vi "AK Befehl Auswerten - AVL Sesam.vi"(10 "Array":string[](array[string])) -> (2 "String für schreiben":string)   [LabVIEW 2020, in "AK-Schnittstelle.lvlib"]
uses:
  AK-Schnittstelle.lvlib
  Aktionen Stoernummern pruefen.ctl
  Aktionen Zustandsfehlerinformation.ctl
  Seiten/FT-IR/FGV FT-IR Diagnose Aktionen.ctl
  Aktionen Gespeicherte Werte.ctl
  Funktionstasten/Funktionstasten-Aktion.ctl
  AK Namen Aktionen.ctl
  Seiten/System Einstellungen V2/Aktioen FGV System.ctl
  EPA 1065/Dichtheitstest 1065-345/Aktion Protokolldaten_Leak check.ctl
  Seiten/FT-IR/Aktion FGV Rezepte wechseln.ctl
  Seiten/FT-IR/FGV FT-IR Aktionen.ctl
  Schedule Modul/Aktion FGV Scheduler Status.ctl
  Seiten/System Einstellungen V2/Aktioen FGV System Konstanten.ctl
  Seiten/FT-IR/AK-manuell.ctl
  Funktionstasten/Zustaende.ctl
  Funktionstasten/Betriebsart.ctl
  EPA 1065/Dichtheitstest 1065-345/Aktion FGV Automatic start.ctl
  Bildwechsel/Bild-Auswahl.ctl
  Seiten/Log Konfig/Aktionen Trigger.ctl
  Seiten/FT-IR/TOOLweb Interface Library/TOOLweb Rezept wechseln.vi
  Funktionstasten/Funktionstasten.lvlib
  Seiten/Log Konfig/LogKonfig.lvlib
  Seiten/FT-IR/FT-IR.lvlib
  Seiten/FT-IR/FGV FT-IR Gasliste Aktionen.ctl
  Seiten/Erweiterte Konfig/Erweiterte Konfig.lvlib
  cRIO/PC/Kommunikation mit cRIO.lvlib
  Seiten/System Einstellungen V2/System Einstellungen V2.lvlib
  Allgemein/allgemeine Sub-VIs.lvlib
  Messdaten/Aktionen FGV Messdaten.ctl
  Messdaten/Messdaten.lvlib
  Schedule Modul/Schedule Modul.lvlib
  EPA 1065/Dichtheitstest 1065-345/Dichtheitstest 1065-345.lvlib
  Seiten/FT-IR/TOOLweb Interface Library/TOOLweb Interface.lvlib
  Bildwechsel/Bildwechsel.lvlib
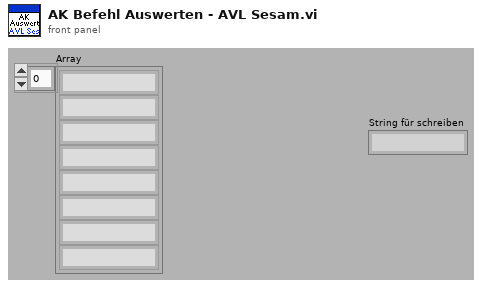
[diagram p1: front panel]
types:
  T1 = typedef "AK-Schnittstelle.lvlib/Aktionen Stoernummern pruefen.ctl" = enum16{"lesen", "prüfen"}
  T2 = typedef "AK-Schnittstelle.lvlib/Aktionen Zustandsfehlerinformation.ctl" = enum16{"OK", "Offline", "Busy", "Syntax Error", "Datenfehler"}
  T3 = typedef "AK-Schnittstelle.lvlib/Aktionen Gespeicherte Werte.ctl" = enum16{"lesen", "laden", "speichern", "Seriell", "TCP", "Diverse", "AKTIV", "AK-Namen"}
  T4 = typedef "FT-IR.lvlib/FGV FT-IR Diagnose Aktionen.ctl" = enum16{"Lesen", "Diagnose Schreiben", "Min Schreiben", "Max Schreiben"}
  T5 = typedef "Funktionstasten.lvlib/Funktionstasten-Aktion.ctl" = enum16{"Initialisieren", "Zustand setzen", "Taste gedrückt", "Fehler speichern", "Lesen", "Manuell", "Remote", "Bitparallel", "Samplepoint", "Zeit Prüfen", "reset Umschalten"}
  T6 = typedef "AK-Schnittstelle.lvlib/AK Namen Aktionen.ctl" = enum16{"lesen", "laden", "speichern Namen", "AK Namen", "Liste erstellen", "EKFG erstellen", "speichern EKFG", "EKFG schreiben", "Neuen Eintrag erzeugen"}
  T7 = typedef "FT-IR.lvlib/FGV FT-IR Gasliste Aktionen.ctl" = enum16{"lesen", "Gasliste FT-IR", "Gasliste ausgelesen", "laden", "speichern", "löschen"}
  T8 = typedef "System Einstellungen V2.lvlib/Aktioen FGV System.ctl" = enum16{"lesen", "laden", "speichern", "Optionen schreiben", "Zeitstempel", "Reset BMP", "Reset SQP", "Wartung", "Werkseinstellung"}
  T9 = typedef "Messdaten.lvlib/Aktionen FGV Messdaten.ctl" = enum16{"lesen", "schreiben", "löschen", "Mittelwerte", "Komponente"}
  T10 = typedef "EPA 1065.lvlib/Dichtheitstest 1065-345.lvlib/Aktion Protokolldaten_Leak check.ctl" = enum16{"lesen", "Zeitstempel", "Bearbeiter", "Daten", "Auswertung", "löschen"}
  T11 = typedef "FT-IR.lvlib/FGV FT-IR Aktionen.ctl" = enum16{"lesen", "NOG setzen", "NOS setzen", "Initialisieren", "speichern", "ALLES setzen", "FT-IR Spektrum loggen", "Komm Stoppen", "Spektrum LogKonfig"}
  T12 = typedef "FT-IR.lvlib/Aktion FGV Rezepte wechseln.ctl" = enum16{"lesen", "Rezepte", "Rezeptindex", "Diesel", "Gasoline", "NCG", "laden", "speichern", "AK/Man"}
  T13 = typedef "Schedule Modul.lvlib/Aktion FGV Scheduler Status.ctl" = enum16{"lesen", "init", "aktiv", "inaktiv"}
  T14 = typedef "System Einstellungen V2.lvlib/Aktioen FGV System Konstanten.ctl" = enum16{"lesen", "laden", "speichern", "Sprache"}
  T15 = typedef "FT-IR.lvlib/AK-manuell.ctl" = enum16{"manuell", "Diesel", "CNG", "Gasoline"}
  T16 = typedef "Funktionstasten.lvlib/Zustaende.ctl" = enum16{"Standby", "Pause", "Eco", "Messen", "Kalibrieren", "Spülen Filter", "Spülen Leitung", "Umgebungsluft", "0-Gas", "Cal-Gas", "CG zu PNS", "-------------", "Init 1", "Init 2", "Init 3", "Init 4", "Messen vorbereiten", "Messen durchführen", "Exit"}
  T17 = typedef "Funktionstasten.lvlib/Betriebsart.ctl" = enum16{"Manuell", "Remote", "Bitparallel"}
  T18 = typedef "EPA 1065.lvlib/Dichtheitstest 1065-345.lvlib/Aktion FGV Automatic start.ctl" = enum16{"lesen", "Test starten aktiv", "Test starten inaktiv", "Seite merken", "Seite zurücksetzen", "AK Start inaktiv"}
  T19 = typedef "Bildwechsel.lvlib/Bild-Auswahl.ctl" = enum16{"lesen", "Initialisieren", "Beenden", "Grafik", "Anlagenübersicht", "Anlagengrenzwerte", "Log Konfig", "Gaszuordnung AO", "Erw. Konfiguration", "FT-IR  ", "Störmeldungen", "Störmeldepuffer", "Störmeldekonfig", "PNS Grenzwerte", "Statusübersicht", "Linearisierung", "ARN", "EPA Dichtheitstest", "FID", "PMA", "CalGas", "Lambda", "Interference", "Amium PNS", "EPA T90", "Interference N2O", "Scheduler", "Systemeinstellungen", "EPA Drift", "CAN Konfig"}
  T20 = typedef "LogKonfig.lvlib/Aktionen Trigger.ctl" = enum16{"lesen", "ALLE schreiben", "Trigger prüfen", "Trigger rücksetzen"}
  T21 = typedef "AK-Schnittstelle.lvlib/Diverse gespeicherte Werte.ctl" = cluster{"Kalibriergaseingang":i16, "SamplePoint":i16, "CalGas zu PNS":i16, "Gas-Reihenfolge":i16[], "Zeit 0-Gas":sgl, "Zeit CalGas":sgl, "AK Befehlssatz":T22}
  T22 = typedef "AK-Schnittstelle.lvlib/AK Befehlssatz.ctl" = enum16{"MEXA", "IAG v1.4", "AVL (Puma)", "PEUS"}
  T23 = typedef "Verwaltung - cRIO.lvlib/Analog Eingaenge.ctl" = cluster{"AI0: Durchfluss FT-IR":sgl, "AI1: Druck Ausgang":sgl, "AI2: Umgebungsdruck":sgl, "AI3: Druck FT-IR":sgl, "AI4: Druck CalGas":sgl, "AI5: Reserve":sgl, "AI6: Reserve":sgl, "AI7: Reserve":sgl, "Rohwert Durchfluss FT-IR":sgl, "Rohwert Druck Ausgang":sgl, "Rohwert Umgebungsdruck":sgl, "Rohwert Druck FT-IR":sgl, "Rohwert Druck CalGas":sgl, "Rohwert AI5":sgl, "Rohwert AI6":sgl, "Rohwert AI7":sgl, "Rohwert Diffdruck mbar FTIR":sgl}
  T24 = typedef "String - Ausgabefeld.ctl" = string
  T25 = typedef "System Einstellungen V2.lvlib/Optionen.ctl" = cluster{"Störmeldep.":bool, "Betriebszustände":bool, "AK in ppm":bool, "log Cal-Gas":bool, "log 0-Gas":bool, "Durchflusssensor 0-5V":bool, "PNS?":bool, "Mit N2 spülen":bool, "TRE08":bool, "Amium 10-Fach":bool, "Verticale Scrollbar aktiv":bool, "Loggingtakt":bool, "AK Rezeptwechsel gleich wie MKS":bool, "NG ECO":bool}
  T26 = typedef "EPA 1065.lvlib/Dichtheitstest 1065-345.lvlib/Leak Daten.ctl" = cluster{"Gesamtes Volumen":sgl, "p 1":sgl, "p 2":sgl, "T 1":sgl, "T 2":sgl, "t 1":timestamp, "t 2":timestamp, "Ergebnis mol/s":sgl, "Grenze mol/s":sgl, "Leak in %":sgl, "Ergebnis mbar":sgl, "Grenze mbar":sgl}
  T27 = typedef "Verwaltung - cRIO.lvlib/TC Eingaenge.ctl" = cluster{"TC0: Reserve":sgl, "TC1: HL zu FT-IR":sgl, "TC2: HL Extern SP1":sgl, "TC3: HL Extern SP2":sgl, "TC4: Reserve":sgl, "TC5: Reserve":sgl, "TC6: Reserve":sgl, "TC7: Reserve":sgl, "TC8: FT-IR":sgl, "TC9: Reserve":sgl, "TC10: Schaltschrank":sgl, "TC11: Umgebung":sgl}
  T28 = cluster{"Modell":string, "ProjektNummer":string, "Software Version":string, "Seriennummer":string}
  T29 = typedef "LogKonfig.lvlib/Element Triggerereignisse.ctl" = cluster{"Trigger verwenden":T30, "Messwert":u16, "kl./gr.":u16, "Wert":sgl, "Puffergröße":sgl}
  T30 = typedef "LogKonfig.lvlib/Auswahlfeld aktiviert-deaktiviert.ctl" = u16
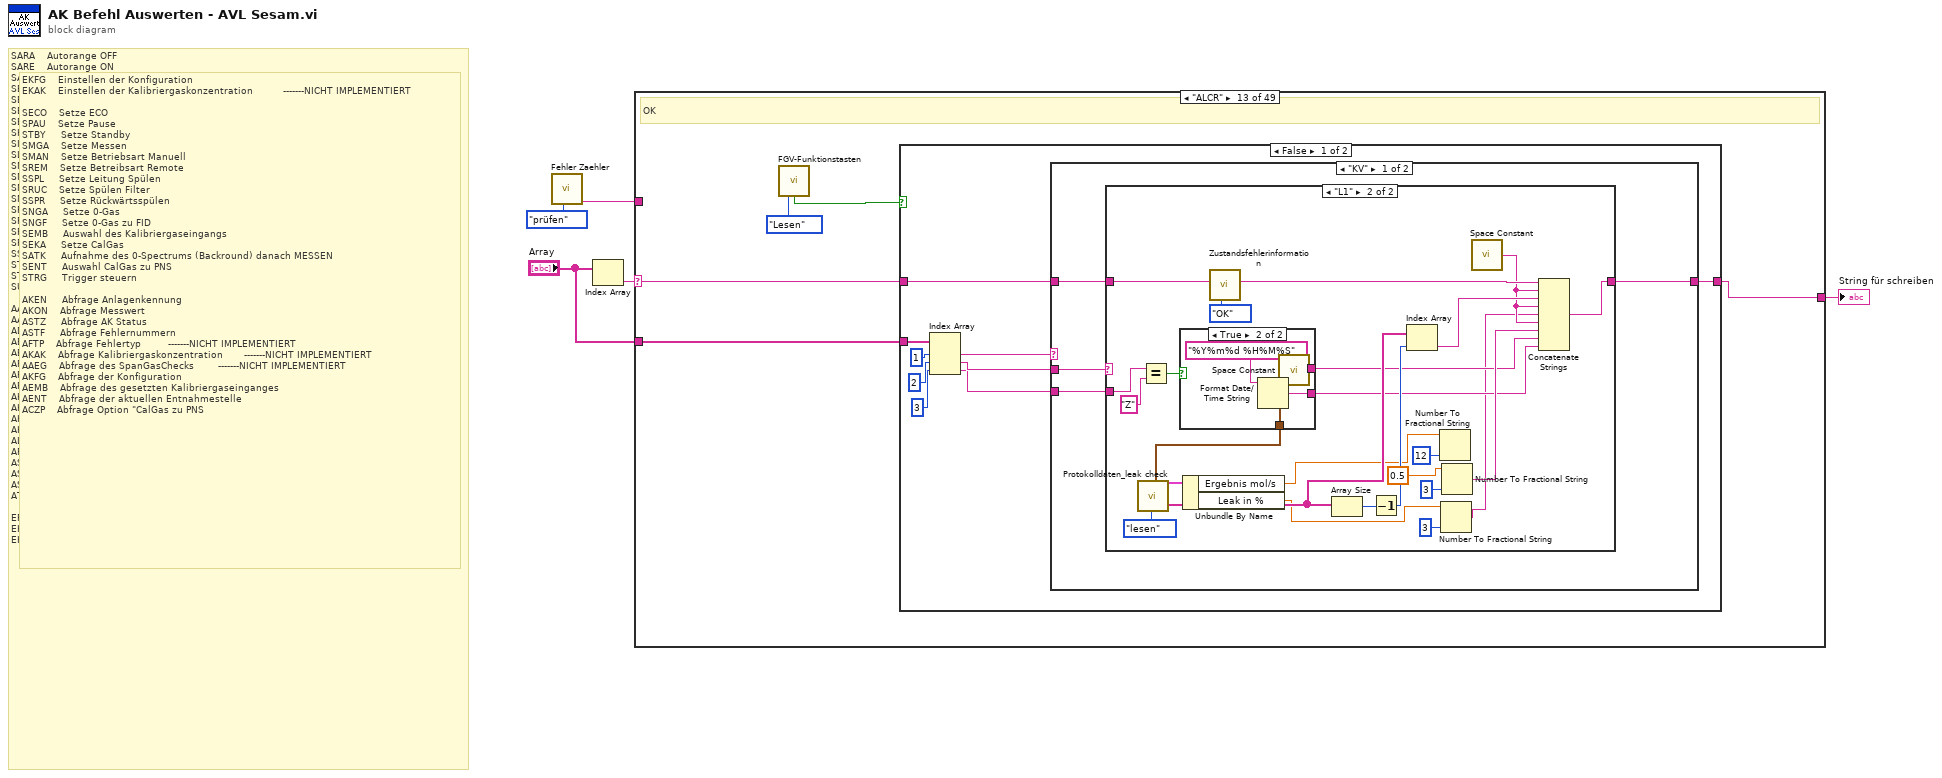
[diagram p0: block diagram]
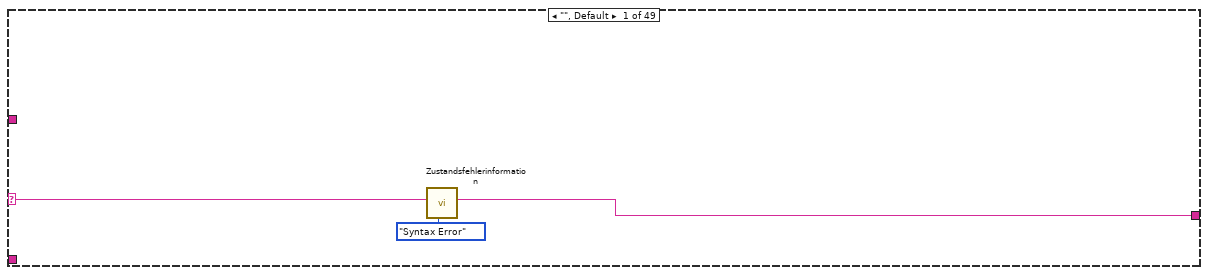
[diagram p2: hidden frame]
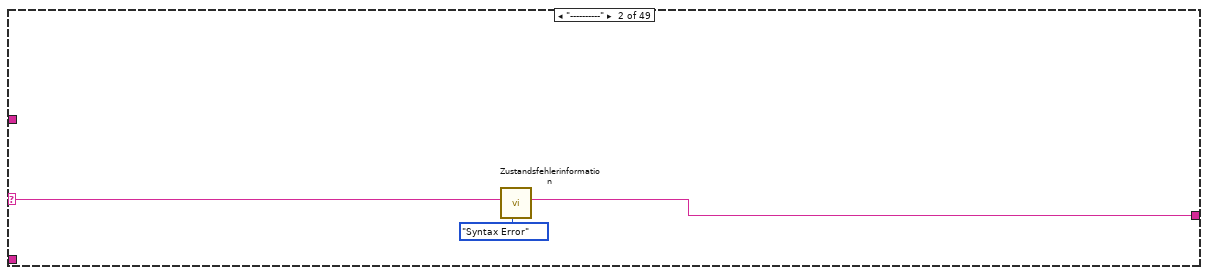
[diagram p3: hidden frame]
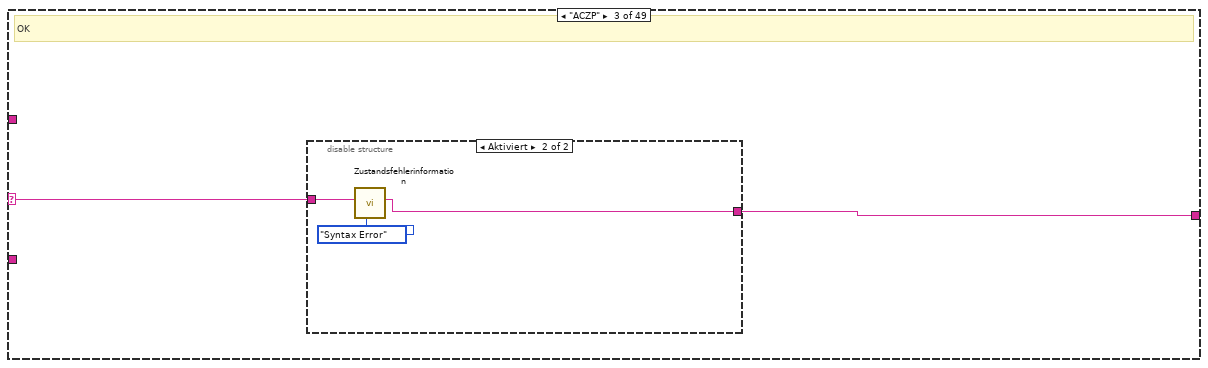
[diagram p4: hidden frame]
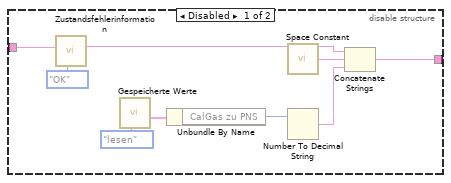
[diagram p5: hidden frame]
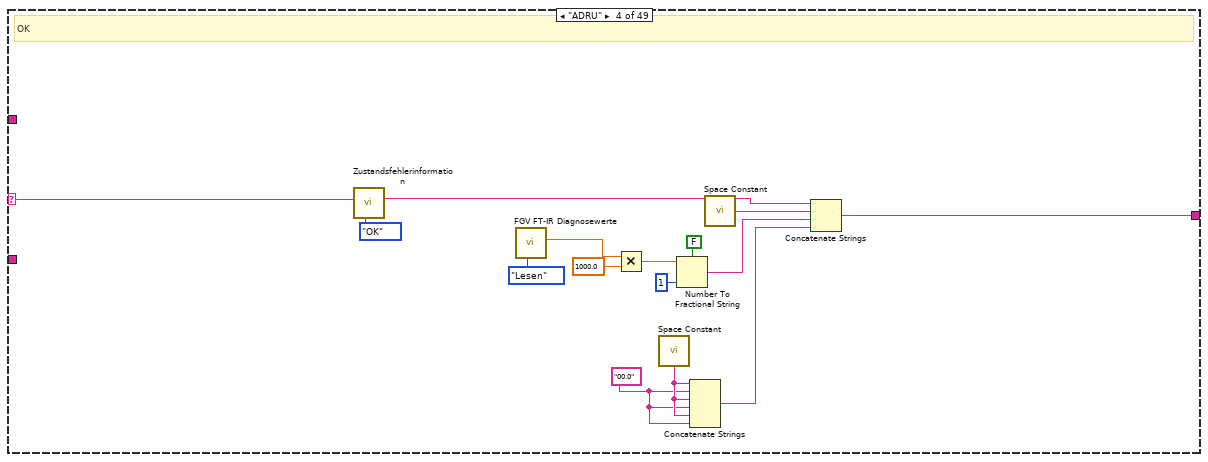
[diagram p6: hidden frame]
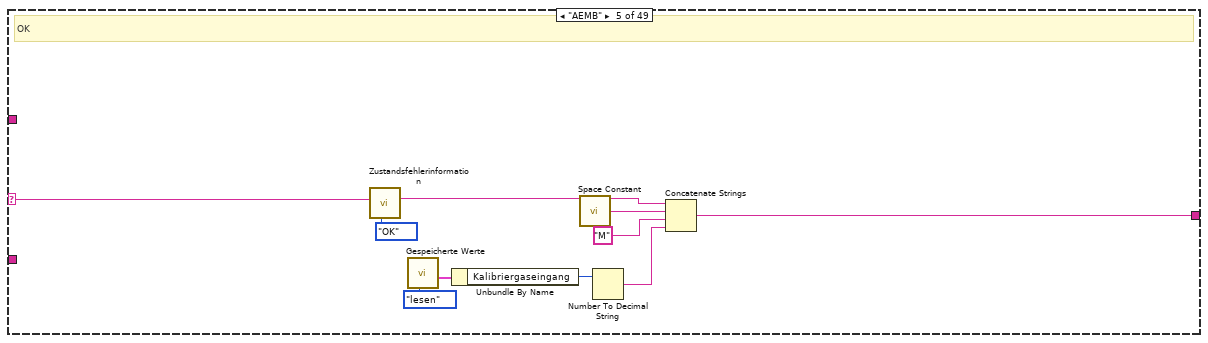
[diagram p7: hidden frame]
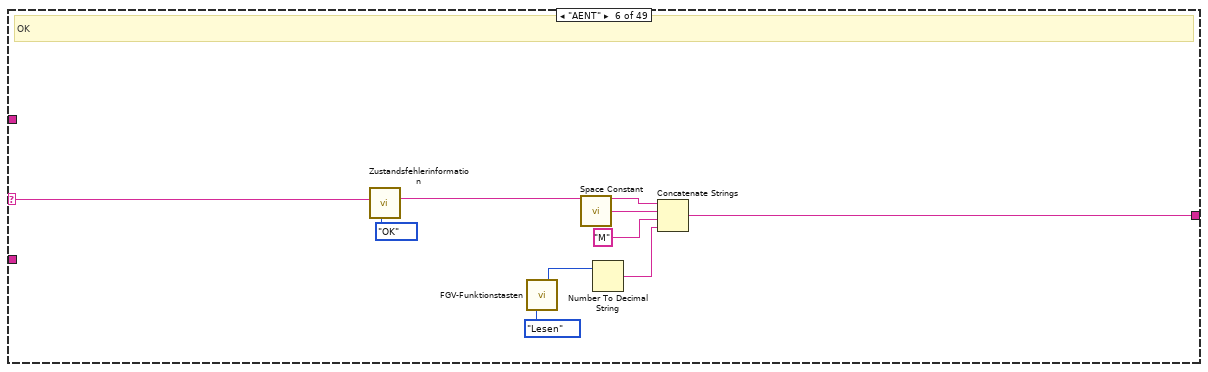
[diagram p8: hidden frame]
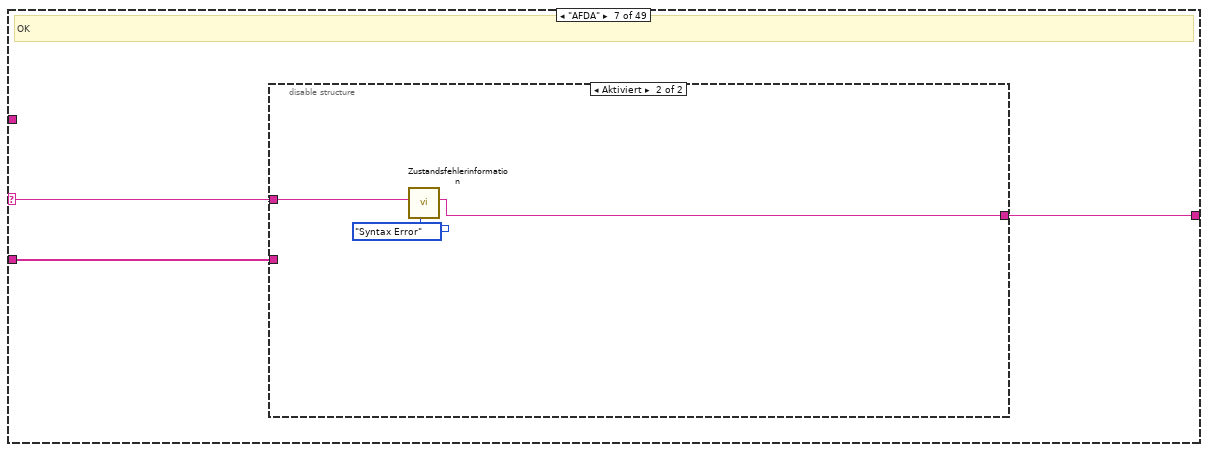
[diagram p9: hidden frame]
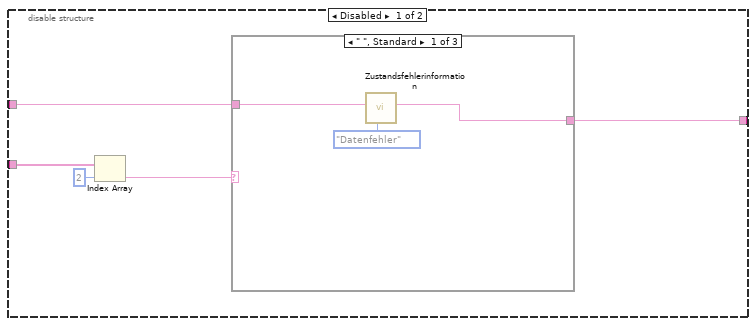
[diagram p10: hidden frame]
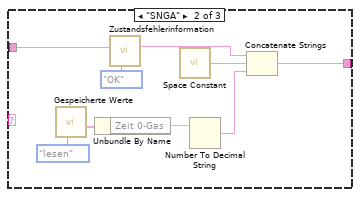
[diagram p11: hidden frame]
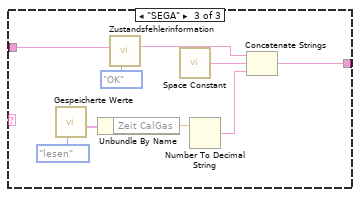
[diagram p12: hidden frame]
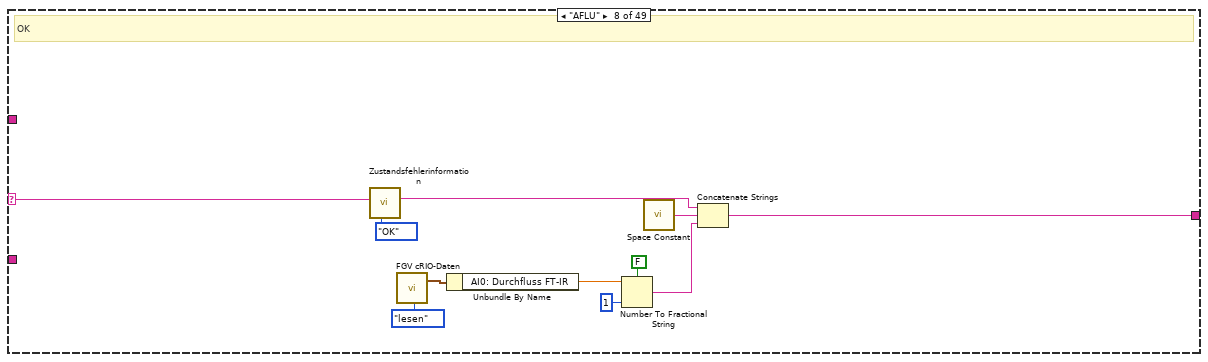
[diagram p13: hidden frame]
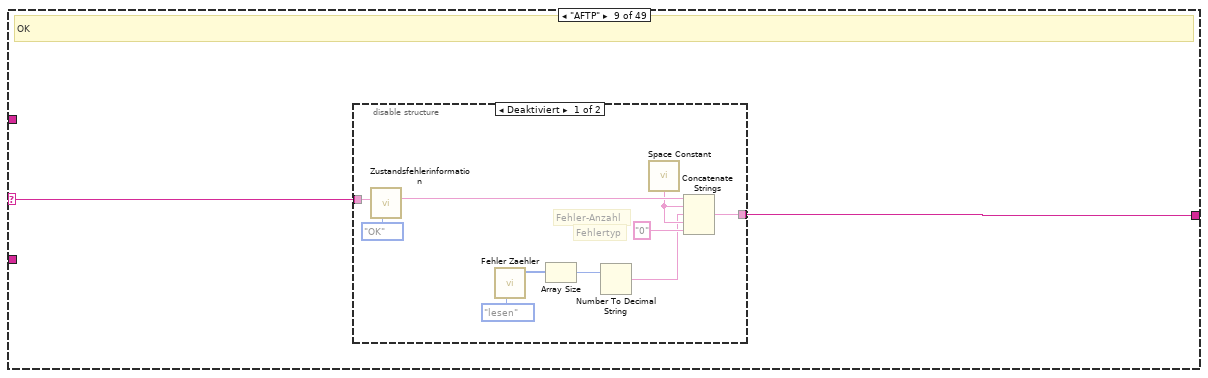
[diagram p14: hidden frame]
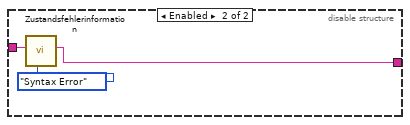
[diagram p15: hidden frame]
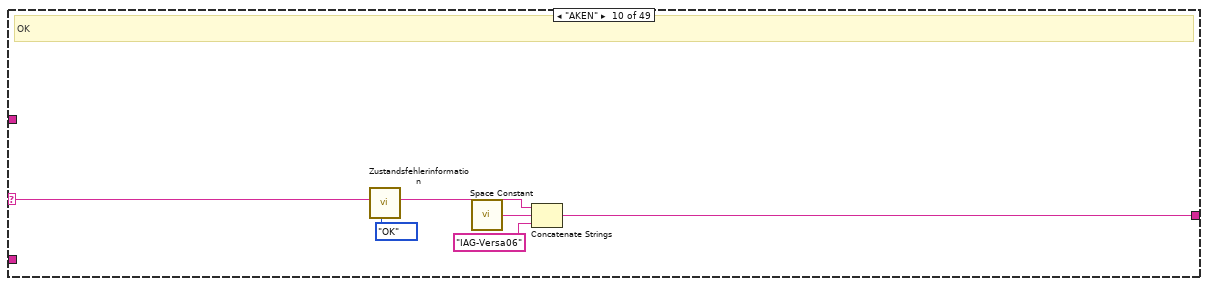
[diagram p16: hidden frame]
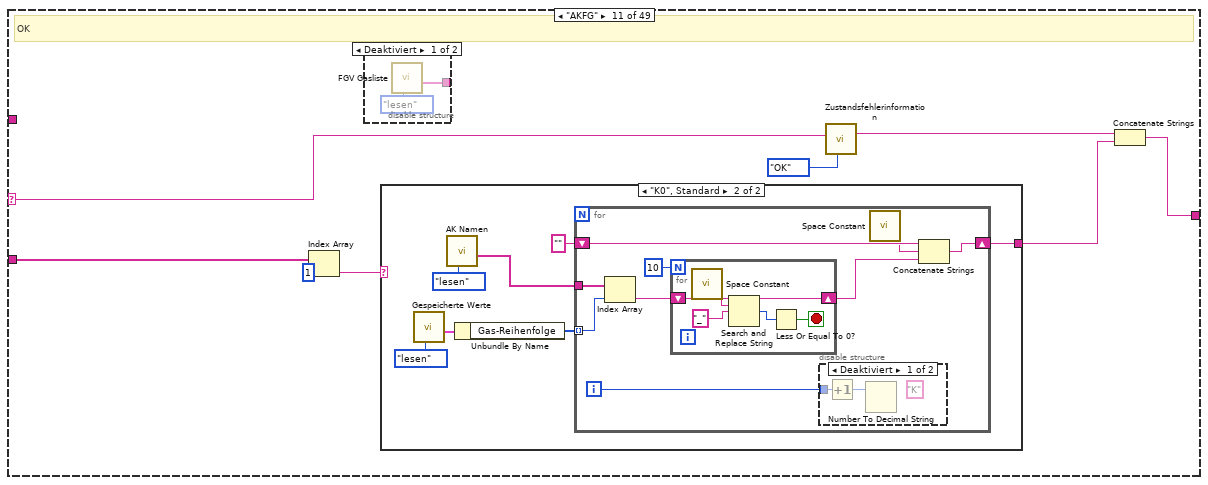
[diagram p17: hidden frame]
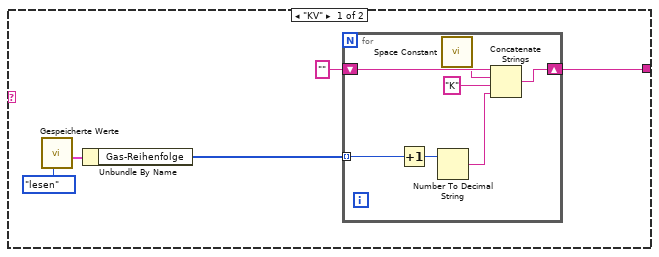
[diagram p18: hidden frame]
diagram:
  # "SARA    Autorange OFF\nSARE    Autorange ON\nSATK    Zero / Span Adjust\nSEGA    Apply Span Gas\nSEKA    Performing FTIR Span Gas Check\nSEMB    Selecting Calibration Gas Inlet\nSENT    Set Sampling\nSHUP    Hang-Up Test         -------NICHT IMPLEMENTIERT\nSINT     Starting Continous FTIR Measurement\nSLEC     Leak Check\nSMAN    Set Manual\nSMGA    Set Measure\nSNGA    Apply Zero Gas\nSNKA    Adjust Zero Point\nSPAU    Pause Modus\nSREM    Set Remote\nSRES    Set Reset\nSRUC / SRUK  Backflush\nSSPL     Purge Gas Lines\nSTBY    Set Standby\nSTUN    Automatically Adjusting Optics and Signals         -------NICHT IMPLEMENTIERT\nSUGR    Recording Zero Energy Spectrum\n\nAAEG    Inquire Span Point Deviation\nAANG    Inquire Zero Point Deviation\nADRU    Inquire Pressure of SESAM FTIR\nAENT    Inquire Sampling Points\nAEMB    Inquire Measuring Range\nAFDA    Inquire Function Duration\nAFLU     Inquire Sample Flow of SBEAM FTIR\nAFTP     Inquire Error Type\nAHUP    Inquire Hangup Result         -------NICHT IMPLEMENTIERT\nAKAK    Inquire Span Gas Concentrations         -------NICHT IMPLEMENTIERT\nAKFG    Inquire Configuration\nAKON   Inquire Measuring Value\nALEC    Inquire Leak Check Result         -------NICHT IMPLEMENTIERT\nAREG    Inquire Control Variable of SESAM FTIR          -------NICHT IMPLEMENTIERT\nASTA    Inquire Erroneous Channel         -------NICHT IMPLEMENTIERT\nASTF    Inquire Error Numbers\nASTZ    Inquire AK Status\nATEM   Inquire Temperature of SESAM FTIR\n\nEFDA   Configure Function Duration\nEKAK   Configure Span Gas Concentration         -------NICHT IMPLEMENTIERT\nEKFG   Configure Configuration"
  # "EKFG    Einstellen der Konfiguration\nEKAK    Einstellen der Kalibriergaskonzentration          -------NICHT IMPLEMENTIERT\n\nSECO    Setze ECO\nSPAU    Setze Pause\nSTBY     Setze Standby\nSMGA    Setze Messen\nSMAN    Setze Betriebsart Manuell\nSREM    Setze Betreibsart Remote\nSSPL     Setze Leitung Spülen\nSRUC    Setze Spülen Filter\nSSPR     Setze Rückwärtsspülen\nSNGA     Setze 0-Gas\nSNGF     Setze 0-Gas zu FID\nSEMB     Auswahl des Kalibriergaseingangs\nSEKA     Setze CalGas\nSATK     Aufnahme des 0-Spectrums (Backround) danach MESSEN\nSENT     Auswahl CalGas zu PNS\nSTRG     Trigger steuern\n\nAKEN     Abfrage Anlagenkennung\nAKON    Abfrage Messwert\nASTZ     Abfrage AK Status\nASTF     Abfrage Fehlernummern\nAFTP    Abfrage Fehlertyp         -------NICHT IMPLEMENTIERT\nAKAK    Abfrage Kalibriergaskonzentration       -------NICHT IMPLEMENTIERT\nAAEG    Abfrage des SpanGasChecks        -------NICHT IMPLEMENTIERT\nAKFG    Abfrage der Konfiguration\nAEMB    Abfrage des gesetzten Kalibriergaseinganges\nAENT    Abfrage der aktuellen Entnahmestelle\nACZP    Abfrage Option \"CalGas zu PNS"
  n1 = call "Fehler Zaehler.vi"("Aktionen"=Aktionen_Stoernummern_pruefen."prüfen") -> ("Fehlerzähler"=w3:string)  [unwired: 7 in, 3 out]
  n2 = Index Array(array="Array") -> (element=w2:string)  [unwired: 1 in]
  n3 = case shown="\"ALCR\"" w2 {
    selector: w2 -> [w7 w10 w12 w38 w48 w57 w61 w100 w103 w120 w129 w189 w245 w317 w321 w342 w349 w367 w407 w432 w437 w475 w506 w541 w544 w547 w551 w553 w567 w571 w593 w620 w623 w659 w662 w676 w679 w683 w685 w689 w691 w695 w706 w716 w726 w730 w733 w736 w758]
    tunnel: [w6 w9 w13 w40 w50 w59 w62 w102 w104 w122 w131 w190 w242 w319 w320 w344 w351 w365 w409 w434 w436 w474 w505 w540 w543 w546 w550 w552 w566 w570 w592 w619 w622 w658 w661 w675 w678 w682 w684 w688 w690 w694 w705 w715 w725 w729 w732 w735 w757] -> w5
    tunnel: w3 -> [_ _ _ _ _ _ _ _ _ _ _ _ _ _ _ _ _ _ _ _ _ _ _ _ _ _ _ _ _ _ _ _ _ _ _ _ _ _ _ _ _ _ _ _ _ _ _ _ _]
    tunnel: "Array" -> [_ _ _ _ _ _ w60 _ _ _ w126 w183 w241 _ _ _ _ w366 _ _ w435 w476 w507 _ _ _ _ _ _ w569 w591 _ w630 _ _ _ _ _ _ _ _ _ w698 w707 w718 _ _ w734 _]
    frame "", Default {
      n4 = call "Zustandsfehlerinformation.vi"("Aktionen"=Aktionen_Zustandsfehlerinformation."Syntax Error", "String"=w7) -> ("String"=w6:string)  [unwired: 9 in]
    }
    frame "----------" {
      n5 = call "Zustandsfehlerinformation.vi"("Aktionen"=Aktionen_Zustandsfehlerinformation."Syntax Error", "String"=w10) -> ("String"=w9:string)  [unwired: 9 in]
    }
    frame "ACZP" {
      # "OK"
      n6 = disable-structure shown="Aktiviert" {
        disable-tunnel: [w22 w23] -> w13
        disable-tunnel: w12 -> [w20 w24]
        frame Disabled {
          n7 = call "Zustandsfehlerinformation.vi"("Aktionen"=Aktionen_Zustandsfehlerinformation."OK", "String"=w20) -> ("String"=w19:string)  [unwired: 9 in]
          n8 = call "Gespeicherte Werte.vi"("Aktionen"=Aktionen_Gespeicherte_Werte."lesen") -> ("Diverse Werte"=w14:T21)  [unwired: 6 in, 4 out]
          n9 = Unbundle By Name(w14) -> ("CalGas zu PNS"=w17:i16)
          n10 = call <vilib>:"Space Constant.vi"() -> ("String"=w15:string)
          n11 = Number To Decimal String(number=w17) -> (decimal integer string=w16:string)  [unwired: 1 in]
          n12 = Concatenate Strings(w19, w15, w16) -> (w22:string)
        }
        frame Enabled {
          n13 = call "Zustandsfehlerinformation.vi"("Aktionen"=Aktionen_Zustandsfehlerinformation."Syntax Error", "String"=w24) -> ("String"=w23:string)  [unwired: 9 in]
        }
      }
    }
    frame "ADRU" {
      w27 = "00.0" ("String in F-Format")
      # "OK"
      n14 = call "Zustandsfehlerinformation.vi"("Aktionen"=Aktionen_Zustandsfehlerinformation."OK", "String"=w38) -> ("String"=w37:string)  [unwired: 9 in]
      n15 = call "FGV FT-IR Diagnosewerte.vi"("Aktionen"=FGV_FT-IR_Diagnose_Aktionen."Lesen") -> ("Druck"=w34:dbl)  [unwired: 5 in, 5 out]
      n16 = Multiply(x=w34, y=1000.0) -> (x*y=w31:dbl)
      n17 = call <vilib>:"Space Constant.vi"() -> ("String"=w28:string)
      n18 = Number To Fractional String(use system decimal point (T)=FALSE ("Systemdezimalzeichen verwenden (T)"), number=w31, precision (6)=i16 1 ("Genauigkeit (6)")) -> (F-format string=w29:string)  [unwired: 1 in]
      n19 = Concatenate Strings(w28, w27, w28, w27, w28, w27) -> (w26:string)
      n20 = call <vilib>:"Space Constant.vi"() -> ("String"=w36:string)
      n21 = Concatenate Strings(w37, w36, w29, w26) -> (w40:string)
    }
    frame "AEMB" {
      # "OK"
      n22 = call "Zustandsfehlerinformation.vi"("Aktionen"=Aktionen_Zustandsfehlerinformation."OK", "String"=w48) -> ("String"=w47:string)  [unwired: 9 in]
      n23 = call "Gespeicherte Werte.vi"("Aktionen"=Aktionen_Gespeicherte_Werte."lesen") -> ("Diverse Werte"=w41:T21)  [unwired: 6 in, 4 out]
      n24 = Unbundle By Name(w41) -> ("Kalibriergaseingang"=w45:i16)
      n25 = call <vilib>:"Space Constant.vi"() -> ("String"=w42:string)
      n26 = Number To Decimal String(number=w45) -> (decimal integer string=w43:string)  [unwired: 1 in]
      n27 = Concatenate Strings(w47, w42, "M" ("String"), w43) -> (w50:string)
    }
    frame "AENT" {
      # "OK"
      n28 = call "Zustandsfehlerinformation.vi"("Aktionen"=Aktionen_Zustandsfehlerinformation."OK", "String"=w57) -> ("String"=w56:string)  [unwired: 9 in]
      n29 = call "FGV-Funktionstasten.vi"("Aktion"=Funktionstasten-Aktion."Lesen") -> ("Samplepoint"=w51:u16)  [unwired: 7 in, 7 out]
      n30 = call <vilib>:"Space Constant.vi"() -> ("String"=w53:string)
      n31 = Number To Decimal String(number=w51) -> (decimal integer string=w54:string)  [unwired: 1 in]
      n32 = Concatenate Strings(w56, w53, "M" ("String"), w54) -> (w59:string)
    }
    frame "AFDA" {
      # "OK"
      n33 = disable-structure shown="Aktiviert" {
        disable-tunnel: [w67 w89] -> w62
        disable-tunnel: w61 -> [w66 w90]
        disable-tunnel: w60 -> [w65 _]
        frame Disabled {
          n34 = Index Array(array=w65, index=2 ("Index")) -> (element=w63:string)
          n35 = case shown="\" \", Standard" w63 {
            tunnel: [w68 w79 w88] -> w67
            tunnel: w66 -> [w69 w77 w86]
            frame " ", Default {
              n36 = call "Zustandsfehlerinformation.vi"("Aktionen"=Aktionen_Zustandsfehlerinformation."Datenfehler", "String"=w69) -> ("String"=w68:string)  [unwired: 9 in]
            }
            frame "SNGA" {
              n37 = call "Gespeicherte Werte.vi"("Aktionen"=Aktionen_Gespeicherte_Werte."lesen") -> ("Diverse Werte"=w74:T21)  [unwired: 6 in, 4 out]
              n38 = Unbundle By Name(w74) -> ("Zeit 0-Gas"=w72:sgl)
              n39 = call "Zustandsfehlerinformation.vi"("Aktionen"=Aktionen_Zustandsfehlerinformation."OK", "String"=w77) -> ("String"=w76:string)  [unwired: 9 in]
              n40 = call <vilib>:"Space Constant.vi"() -> ("String"=w75:string)
              n41 = Number To Decimal String(number=w72) -> (decimal integer string=w71:string)  [unwired: 1 in]
              n42 = Concatenate Strings(w76, w75, w71) -> (w79:string)
            }
            frame "SEGA" {
              n43 = call "Gespeicherte Werte.vi"("Aktionen"=Aktionen_Gespeicherte_Werte."lesen") -> ("Diverse Werte"=w83:T21)  [unwired: 6 in, 4 out]
              n44 = Unbundle By Name(w83) -> ("Zeit CalGas"=w81:sgl)
              n45 = call "Zustandsfehlerinformation.vi"("Aktionen"=Aktionen_Zustandsfehlerinformation."OK", "String"=w86) -> ("String"=w85:string)  [unwired: 9 in]
              n46 = call <vilib>:"Space Constant.vi"() -> ("String"=w84:string)
              n47 = Number To Decimal String(number=w81) -> (decimal integer string=w80:string)  [unwired: 1 in]
              n48 = Concatenate Strings(w85, w84, w80) -> (w88:string)
            }
          }
        }
        frame Enabled {
          n49 = call "Zustandsfehlerinformation.vi"("Aktionen"=Aktionen_Zustandsfehlerinformation."Syntax Error", "String"=w90) -> ("String"=w89:string)  [unwired: 9 in]
        }
      }
    }
    frame "AFLU" {
      # "OK"
      n50 = call "Zustandsfehlerinformation.vi"("Aktionen"=Aktionen_Zustandsfehlerinformation."OK", "String"=w100) -> ("String"=w99:string)  [unwired: 9 in]
      n51 = call "FGV cRIO-Daten.vi"("Aktion"=enum16{"lesen", "schreiben"}."lesen") -> ("Analog Input"=w96:T23)  [unwired: 9 in, 9 out]
      n52 = Unbundle By Name(w96) -> ("AI0: Durchfluss FT-IR"=w93:sgl)
      n53 = Number To Fractional String(use system decimal point (T)=FALSE ("Systemdezimalzeichen verwenden (T)"), number=w93, precision (6)=i16 1 ("Genauigkeit (6)")) -> (F-format string=w92:string)  [unwired: 1 in]
      n54 = call <vilib>:"Space Constant.vi"() -> ("String"=w98:string)
      n55 = Concatenate Strings(w99, w98, w92) -> (w102:string)
    }
    frame "AFTP" {
      # "OK"
      n56 = disable-structure shown="Deaktiviert" {
        disable-tunnel: [w114 w115] -> w104
        disable-tunnel: w103 -> [w112 w116]
        frame Disabled {
          # "Fehlertyp"
          # "Fehler-Anzahl"
          n57 = call "Zustandsfehlerinformation.vi"("Aktionen"=Aktionen_Zustandsfehlerinformation."OK", "String"=w112) -> ("String"=w111:string)  [unwired: 9 in]
          n58 = call "Fehler Zaehler.vi"("Aktionen"=Aktionen_Stoernummern_pruefen."lesen") -> ("Fehler Nummern"=w109:i32[])  [unwired: 7 in, 3 out]
          n59 = Array Size(array=w109) -> (size(s)=w108:i32)
          n60 = Number To Decimal String(number=w108) -> (decimal integer string=w105:string)  [unwired: 1 in]
          n61 = call <vilib>:"Space Constant.vi"() -> ("String"=w107:string)
          n62 = Concatenate Strings(w111, w107, w105, w107, "0" ("String")) -> (w114:string)
        }
        frame Enabled {
          n63 = call "Zustandsfehlerinformation.vi"("Aktionen"=Aktionen_Zustandsfehlerinformation."Syntax Error", "String"=w116) -> ("String"=w115:string)  [unwired: 9 in]
        }
      }
    }
    frame "AKEN" {
      # "OK"
      n64 = call "Zustandsfehlerinformation.vi"("Aktionen"=Aktionen_Zustandsfehlerinformation."OK", "String"=w120) -> ("String"=w119:string)  [unwired: 9 in]
      n65 = call <vilib>:"Space Constant.vi"() -> ("String"=w118:string)
      n66 = Concatenate Strings(w119, w118, "IAG-Versa06" ("String")) -> (w122:string)
    }
    frame "AKFG" {
      # "OK"
      n67 = Index Array(array=w126, index=1 ("Index")) -> (element=w124:string)
      n68 = disable-structure shown="Deaktiviert" {
        disable-tunnel: [w168 _] -> _
        frame Disabled {
          n69 = call "FGV Gasliste.vi"("Aktionen"=FGV_FT-IR_Gasliste_Aktionen."lesen") -> ("Aktuelle Gasliste gesamt"=w168:T24[])  [unwired: 8 in, 2 out]
        }
        frame Enabled {
        }
      }
      n70 = case shown="\"K0\", Standard" w124 {
        tunnel: [w132 w148] -> w127
        frame "KV" {
          n71 = call "Gespeicherte Werte.vi"("Aktionen"=Aktionen_Gespeicherte_Werte."lesen") -> ("Diverse Werte"=w136:T21)  [unwired: 6 in, 4 out]
          n72 = Unbundle By Name(w136) -> ("Gas-Reihenfolge"=w134:i16[])
          n73 = for {
            tunnel: w134 -> [w139] mode=indexing
            shift-right: [w143] -> w132
            shift-left: "" -> [w142]
            n74 = Increment(x=w139) -> (x+1=w140:i16)
            n75 = Number To Decimal String(number=w140) -> (decimal integer string=w137:string)  [unwired: 1 in]
            n76 = call <vilib>:"Space Constant.vi"() -> ("String"=w141:string)
            n77 = Concatenate Strings(w142, w141, "K" ("String"), w137) -> (w143:string)
          }
        }
        frame "K0", Default {
          n78 = call "Gespeicherte Werte.vi"("Aktionen"=Aktionen_Gespeicherte_Werte."lesen") -> ("Diverse Werte"=w146:T21)  [unwired: 6 in, 4 out]
          n79 = call "AK Namen.vi"("Aktionen"=AK_Namen_Aktionen."lesen") -> ("AK Namen"=w144:string[])  [unwired: 7 in, 3 out]
          n80 = Unbundle By Name(w146) -> ("Gas-Reihenfolge"=w149:i16[])
          n81 = for {
            tunnel: w149 -> [w156] mode=indexing
            shift-right: [w159] -> w148
            shift-left: "" -> [w158]
            tunnel: w144 -> [w157]
            i -> [w151]
            n82 = Index Array(array=w157, index=w156) -> (element=w154:string)
            n83 = for {
              N: 10 -> [_]
              shift-right: [w166] -> w153
              shift-left: w154 -> [w167]
              stop <- w164 stop-if-true
              n84 = call <vilib>:"Space Constant.vi"() -> ("String"=w163:string)
              n85 = Search and Replace String(input string=w167, search string=w163, replace string="_") -> (result string=w166:string, number of replacements=w165:i32)  [unwired: 5 in, 2 out]
              n86 = Less Or Equal To 0?(x=w165) -> (x <= 0?=w164:bool)
            }
            n87 = disable-structure shown="Deaktiviert" {
              disable-tunnel: w151 -> [w160 _]
              frame Disabled {
                (unwired) "K" ("String")
                n88 = Increment(x=w160) -> (x+1=w161:i32)
                n89 = Number To Decimal String(number=w161) -> ()  [unwired: 1 in, 1 out]
              }
              frame Enabled {
              }
            }
            n90 = call <vilib>:"Space Constant.vi"() -> ("String"=w152:string)
            n91 = Concatenate Strings(w158, w152, w153) -> (w159:string)
          }
        }
      }
      n92 = call "Zustandsfehlerinformation.vi"("Aktionen"=Aktionen_Zustandsfehlerinformation."OK", "String"=w129) -> ("String"=w128:string)  [unwired: 9 in]
      n93 = Concatenate Strings(w128, w127) -> (w131:string)
    }
    frame "AKON" {
      # "OK"
      n94 = call "FGV System.vi"("Aktionen"=Aktioen_FGV_System."lesen") -> ("Optionen"=w174:T25)  [unwired: 12 in, 6 out]
      n95 = Unbundle By Name(w174) -> ("AK in ppm"=w171:bool)
      n96 = disable-structure shown="Aktiviert" {
        disable-tunnel: [w192 w194] -> w170
        frame Disabled {
          n97 = call "FGV Messdaten.vi"("Aktionen"=Aktionen_FGV_Messdaten."lesen") -> ("Aktuelle Messwerte"=w192:sgl[])  [unwired: 6 in, 8 out]
        }
        frame Enabled {
          n98 = call "Rolling Average Umschaltung Anzeige.vi"("Aktion"=enum16{"AK", "IAG Software"}."AK") -> ("Aktuelle Messwerte"=w194:sgl[])  [unwired: 9 in, 5 out]
        }
      }
      n99 = call "Gespeicherte Werte.vi"("Aktionen"=Aktionen_Gespeicherte_Werte."lesen") -> ("Diverse Werte"=w181:T21)  [unwired: 6 in, 4 out]
      n100 = Index Array(array=w183, index=1 ("Index")) -> (element=w178:string)
      n101 = Unbundle By Name(w181) -> ("Gas-Reihenfolge"=w186:i16[])
      n102 = case shown="True" w171 {
        tunnel: w170 -> [w195 w197]
        tunnel: [w195 w196] -> w172
        frame False {
        }
        frame True {
          n103 = call "H2O und CO2 umrechnen.vi"("Aktuelle Messwerte"=w197) -> ("Aktuelle Messwerte"=w196:sgl[])  [unwired: 10 in]
        }
      }
      n104 = Equal?(x=w178, y="K0") -> (x = y?=w177:bool)
      n105 = Equal?(x=w178, y="KV") -> (x = y?=w176:bool)
      n106 = Or(x=w177, y=w176) -> (x .or. y?=w175:bool)
      n107 = case shown="False" w175 {
        tunnel: w186 -> [w200 w232]
        tunnel: [w198 w230] -> w185
        tunnel: w172 -> [w199 w229]
        tunnel: w183 -> [w204 _]
        tunnel: [w202 Aktionen_Zustandsfehlerinformation."OK" ("Aktionen")] -> w182
        frame False {
          n108 = Delete From Array(array=w204, length=1 ("Länge"), index=0 ("Index")) -> (array with subset deleted=w201:string[])  [unwired: 1 out]
          n109 = Empty Array?(array=w201) -> (empty?=w203:bool)
          n110 = case shown="False" w203 {
            tunnel: [Aktionen_Zustandsfehlerinformation."OK" ("Aktionen") Aktionen_Zustandsfehlerinformation."Datenfehler" ("Aktionen")] -> w202
            tunnel: w201 -> [w211 _]
            tunnel: w200 -> [w210 _]
            tunnel: w199 -> [w209 _]
            tunnel: [w208 ""] -> w198
            frame False {
              # "Je nach Abgefragten Kanal den RICHTIGEN\nMesswert heraussuchen!"
              n111 = for {
                tunnel: w211 -> [w225] mode=indexing
                tunnel: w210 -> [w223]
                tunnel: w209 -> [w222]
                shift-right: [w221] -> w208
                shift-left: "" -> [w218]
                n112 = Decimal String To Number(string=w225, offset=1 ("Offset (0)")) -> (number=w217:i32)  [unwired: 1 in, 1 out]
                n113 = Decrement(x=w217) -> (x-1=w216:i32)
                n114 = Index Array(array=w223, index=w216) -> (element=w214:i16)
                n115 = Index Array(array=w222, index=w214) -> (element=w220:sgl)
                n116 = call <vilib>:"Space Constant.vi"() -> ("String"=w215:string)
                n117 = Number To Fractional String(use system decimal point (T)=FALSE ("Systemdezimalzeichen verwenden (T)"), number=w220) -> (F-format string=w219:string)  [unwired: 2 in]
                n118 = Concatenate Strings(w218, w215, w219) -> (w221:string)
              }
            }
            frame True {
              # "Wenn der String leer ist, dann Datenfehler"
            }
          }
        }
        frame True {
          n119 = for {
            tunnel: w232 -> [w234] mode=indexing
            shift-right: [w240] -> w230
            shift-left: "" -> [w239]
            tunnel: w229 -> [w238]
            n120 = Index Array(array=w238, index=w234) -> (element=w237:sgl)
            n121 = Number To Fractional String(use system decimal point (T)=FALSE ("Systemdezimalzeichen verwenden (T)"), number=w237) -> (F-format string=w236:string)  [unwired: 2 in]
            n122 = call <vilib>:"Space Constant.vi"() -> ("String"=w235:string)
            n123 = Concatenate Strings(w239, w235, w236) -> (w240:string)
          }
        }
      }
      n124 = call "Zustandsfehlerinformation.vi"("Aktionen"=w182, "String"=w189) -> ("String"=w188:string)  [unwired: 9 in]
      n125 = Concatenate Strings(w188, w185) -> (w190:string)
    }
    frame "ALCR" {
      # "OK"
      n126 = call "FGV-Funktionstasten.vi"("Aktion"=Funktionstasten-Aktion."Lesen") -> ("Busy"=w243:bool)  [unwired: 7 in, 7 out]
      n127 = case shown="False" w243 {
        tunnel: w245 -> [w254 w295]
        tunnel: [w251 w294] -> w242
        tunnel: w241 -> [w252 _]
        frame False {
          n128 = Index Array(array=w252, index #1=1 ("Index"), index #2=2 ("Index"), index #3=3 ("Index")) -> (element #1=w250:string, element #2=w248:string, element #3=w246:string)
          n129 = case shown="\"KV\"" w250 {
            tunnel: w254 -> [w258 w292]
            tunnel: [w257 w291] -> w251
            tunnel: w248 -> [w256 _]
            tunnel: w246 -> [w255 _]
            frame "KV" {
              n130 = case shown="\"L1\"" w256 {
                tunnel: w258 -> [w260 w286]
                tunnel: [w259 w284] -> w257
                tunnel: w255 -> [_ w285]
                frame "False", Default {
                  n131 = call "Zustandsfehlerinformation.vi"("Aktionen"=Aktionen_Zustandsfehlerinformation."Syntax Error", "String"=w260) -> ("String"=w259:string)  [unwired: 9 in]
                }
                frame "L1" {
                  n132 = call "Protokolldaten_leak check.vi"("Aktion"=Aktion_Protokolldaten_Leak_check."lesen") -> ("Start"=w280:timestamp, "Auswertung"=w278:string[], "Daten"=w264:T26)  [unwired: 23 in, 1 out]
                  n133 = Equal?(x=w285, y="Z") -> (x = y?=w276:bool)
                  n134 = case shown="True" w276 {
                    tunnel: w280 -> [_ w290]
                    tunnel: [_ w288] -> w268
                    tunnel: [_ w287] -> w269
                    frame False {
                    }
                    frame True {
                      n135 = Format Date/Time String(time format string (%c)="%Y%m%d %H%M%S" ("Zeitformatierungs-String (%c)"), seconds (now)=w290) -> (date/time string=w288:string)  [unwired: 1 in]
                      n136 = call <vilib>:"Space Constant.vi"() -> ("String"=w287:string)
                    }
                  }
                  n137 = Unbundle By Name(w264) -> ("Ergebnis mol/s"=w263:sgl, "Leak in %"=w262:sgl)
                  n138 = call "Zustandsfehlerinformation.vi"("Aktionen"=Aktionen_Zustandsfehlerinformation."OK", "String"=w286) -> ("String"=w273:string)  [unwired: 9 in]
                  n139 = Array Size(array=w278) -> (size(s)=w279:i32)
                  n140 = Decrement(x=w279) -> (x-1=w277:i32)
                  n141 = Index Array(array=w278, index=w277) -> (element=w272:string)
                  n142 = Number To Fractional String(number=w263, precision (6)=i16 12 ("Genauigkeit (6)")) -> ()  [unwired: 2 in, 1 out]
                  n143 = Number To Fractional String(number=w262, precision (6)=i16 3 ("Genauigkeit (6)")) -> (F-format string=w266:string)  [unwired: 2 in]
                  n144 = Number To Fractional String(number=0.5 ("Zahl"), precision (6)=i16 3 ("Genauigkeit (6)")) -> (F-format string=w271:string)  [unwired: 2 in]
                  n145 = call <vilib>:"Space Constant.vi"() -> ("String"=w270:string)
                  n146 = Concatenate Strings(w273, w270, w272, w270, w266, w270, w271, w269, w268) -> (w284:string)
                }
              }
            }
            frame "False", Default {
              n147 = call "Zustandsfehlerinformation.vi"("Aktionen"=Aktionen_Zustandsfehlerinformation."Syntax Error", "String"=w292) -> ("String"=w291:string)  [unwired: 9 in]
            }
          }
        }
        frame True {
          n148 = call "Zustandsfehlerinformation.vi"("Aktionen"=Aktionen_Zustandsfehlerinformation."Busy", "String"=w295) -> ("String"=w294:string)  [unwired: 9 in]
        }
      }
    }
    frame "AMET" {
      # "OK"
      n149 = call "FGV Rezepte wechseln.vi"("Aktion"=Aktion_FGV_Rezepte_wechseln."lesen") -> ("Rezepte"=w312:string[], "Diesel"=w310:u16, "Gasoline"=w306:u16, "Natural Gas"=w297:u16)  [unwired: 8 in, 3 out]
      n150 = call "FGV FT-IR Parameter.vi"("Aktion"=FGV_FT-IR_Aktionen."lesen") -> ("Current Recipe"=w311:string)  [unwired: 11 in, 7 out]
      n151 = call "Zustandsfehlerinformation.vi"("Aktionen"=Aktionen_Zustandsfehlerinformation."OK", "String"=w317) -> ("String"=w316:string)  [unwired: 9 in]
      n152 = call "String in Array suchen.vi"("Nach String/Zeichen suchen (-)"=w311, "String-Array"=w312) -> ("Index"=w298:i32)  [unwired: 7 in, 2 out]
      n153 = Equal?(x=w297, y=w298) -> (x = y?=w302:bool)
      n154 = Equal?(x=w306, y=w298) -> (x = y?=w305:bool)
      n155 = Equal?(x=w310, y=w298) -> (x = y?=w309:bool)
      n156 = Select(t="DIESEL", s=w309, f="") -> (s? t:f=w304:string)
      n157 = Select(t="GASOLINE", s=w305, f=w304) -> (s? t:f=w301:string)
      n158 = Select(t="CNG", s=w302, f=w301) -> (s? t:f=w299:string)
      n159 = call <vilib>:"Space Constant.vi"() -> ("String"=w315:string)
      n160 = Concatenate Strings(w316, w315, w299) -> (w319:string)
    }
    frame "ARLT" {
      # "OK"
      n161 = disable-structure shown="Aktiviert" {
        disable-tunnel: w321 -> [w336 w338]
        disable-tunnel: [w335 w338] -> w333
        frame Disabled {
          n162 = call "Zustandsfehlerinformation.vi"("Aktionen"=Aktionen_Zustandsfehlerinformation."OK", "String"=w336) -> ("String"=w335:string)  [unwired: 9 in]
        }
        frame Enabled {
        }
      }
      n163 = call "FGV Rezepte wechseln.vi"("Aktion"=Aktion_FGV_Rezepte_wechseln."lesen") -> ("Rezepte"=w332:string[])  [unwired: 8 in, 6 out]
      n164 = Array To Spreadsheet String(delimiter (Tab)="],[" ("Trennzeichen (Tabulator)"), array=w332, 3:"%s" ("Format-String")) -> (spreadsheet string=w323:string)
      n165 = String Length(string=w323) -> (length=w326:i32)
      n166 = Subtract(x=w326, y=2) -> (x-y=w324:i32)
      n167 = String Subset(string=w323, length (rest)=w324) -> (substring=w328:string)  [unwired: 1 in]
      n168 = call <vilib>:"Space Constant.vi"() -> ("String"=w334:string)
      n169 = Concatenate Strings(w333, w334, "\"[" ("String"), w328, "]\"") -> (w320:string)
    }
    frame "ASTA" {
      # "OK"
      n170 = call "Zustandsfehlerinformation.vi"("Aktionen"=Aktionen_Zustandsfehlerinformation."OK", "String"=w342) -> ("String"=w341:string)  [unwired: 9 in]
      n171 = call <vilib>:"Space Constant.vi"() -> ("String"=w339:string)
      n172 = Concatenate Strings(w341, w339, "KV" ("String")) -> (w344:string)
    }
    frame "ASTF" {
      # "OK"
      n173 = call "Zustandsfehlerinformation.vi"("Aktionen"=Aktionen_Zustandsfehlerinformation."OK", "String"=w349) -> ("String"=w348:string)  [unwired: 9 in]
      n174 = call "Fehler Zaehler.vi"("Aktionen"=Aktionen_Stoernummern_pruefen."lesen") -> ("Fehler Nummern"=w346:string)  [unwired: 7 in, 3 out]
      n175 = call <vilib>:"Space Constant.vi"() -> ("String"=w345:string)
      n176 = Concatenate Strings(w348, w345, w346) -> (w351:string)
    }
    frame "ASTZ" {
      # "OK"
      n177 = Index Array(array=w366, index=1 ("Index")) -> (element=w359:string)
      n178 = call "Zustandsfehlerinformation.vi"("Aktionen"=Aktionen_Zustandsfehlerinformation."OK", "String"=w367) -> ("String"=w363:string)  [unwired: 9 in]
      n179 = call "FGV Schedule Status.vi"("Aktion"=Aktion_FGV_Scheduler_Status."lesen") -> ("Scheduler Status"=w354:bool)  [unwired: 13 in, 1 out]
      n180 = call "FGV-Funktionstasten.vi"("Aktion"=Funktionstasten-Aktion."Lesen") -> ("ausgewählte Funktion"=w353:T16, "Betriebsart"=w361:T17)  [unwired: 7 in, 6 out]
      n181 = case shown="False" w354 {
        tunnel: w353 -> [w369 _]
        tunnel: [w368 "SATK" ("String")] -> w352
        frame False {
          n182 = case shown="\"Standby\", Standard" w369 {
            tunnel: ["STBY" ("String") "SPAU" ("String") "SECO" ("String") "SMGA" ("String") "SATK" ("String") "SEKA" ("String") "SRUC" ("String") "SSPL" ("String") "SNGA" ("String") "SCZP" ("String") _ _ _ _ _ _ _ _] -> w368
            frame "Standby", Default {
            }
            frame "Pause" {
            }
            frame "Eco" {
            }
            frame "Messen" {
            }
            frame "Kalibrieren" {
            }
            frame "Cal-Gas" {
              # "#KaliAutoMessenBug"
            }
            frame "Spülen Filter" {
            }
            frame "Spülen Leitung" {
            }
            frame "0-Gas" {
            }
            frame "CG zu PNS" {
              # "#KaliAutoMessenBug"
            }
            frame "Init 1" {
            }
            frame "Init 2" {
            }
            frame "-------------" {
            }
            frame "Init 3" {
            }
            frame "Init 4" {
            }
            frame "Messen vorbereiten" {
            }
            frame "Messen durchführen" {
            }
            frame "Exit" {
            }
          }
        }
        frame True {
        }
      }
      n183 = case shown="\"KV\"" w359 {
        selector: w359 -> [w381 _ _]
        tunnel: [w381 "K1" ("String") "KV" ("String")] -> w358
        frame "K1", Default {
        }
        frame "K0" {
        }
        frame "KV" {
        }
      }
      n184 = case shown="\"Remote\"" w361 {
        tunnel: ["SMAN" ("String") "SREM" ("String") "SBIT" ("String")] -> w357
        frame "Manuell", Default {
        }
        frame "Remote" {
        }
        frame "Bitparallel" {
        }
      }
      n185 = call <vilib>:"Space Constant.vi"() -> ("String"=w356:string)
      n186 = Concatenate Strings(w363, w356, w358, w356, w357, w356, w352) -> (w365:string)
      n187 = disable-structure shown="Aktiviert" {
        frame Disabled {
          n188 = Index Array(index=1 ("Index")) -> (element=w388)  [unwired: 1 in]
          n189 = call "Zustandsfehlerinformation.vi"("Aktionen"=Aktionen_Zustandsfehlerinformation."OK") -> (2:"String"=w391:string, 10:"String"=w393:string)  [unwired: 9 in]
          n190 = call "ASTZ - AVL Sesam.vi"("Selektor"=w388) -> ("Verknüpfter String"=w387:string)  [unwired: 10 in]
          n191 = call <vilib>:"Space Constant.vi"() -> ("String"=w389:string)
          n192 = Concatenate Strings(w391, w389, w387) -> ()  [unwired: 1 out]
        }
        frame Enabled {
        }
      }
    }
    frame "ATEM" {
      # "OK"
      n193 = call "FGV cRIO-Daten.vi"("Aktion"=enum16{"lesen", "schreiben"}."lesen") -> ("TC Eingänge"=w398:T27)  [unwired: 9 in, 9 out]
      n194 = Cluster To Array(cluster=w398) -> (array=w397:sgl[])
      n195 = call <vilib>:"Space Constant.vi"() -> ("String"=w395:string)
      n196 = Array Size(array=w397) -> (size(s)=w396:i32)
      n197 = call "Zustandsfehlerinformation.vi"("Aktionen"=Aktionen_Zustandsfehlerinformation."OK", "String"=w407) -> ("String"=w406:string)  [unwired: 9 in]
      n198 = for {
        shift-right: [w413] -> w394
        shift-left: w395 -> [w419]
        tunnel: w397 -> [w415] mode=indexing
        tunnel: w396 -> [w411]
        i -> [w414]
        n199 = Number To Fractional String(use system decimal point (T)=FALSE ("Systemdezimalzeichen verwenden (T)"), number=w415, precision (6)=i16 1 ("Genauigkeit (6)")) -> (F-format string=w416:string)  [unwired: 1 in]
        n200 = Increment(x=w414) -> (x+1=w412:i32)
        n201 = Equal?(x=w411, y=w412) -> (x = y?=w410:bool)
        n202 = case shown="False" w410 {
          tunnel: w419 -> [w422 w426]
          tunnel: w416 -> [w421 w425]
          tunnel: [w420 w423] -> w413
          frame True {
            n203 = Concatenate Strings(w422, w421) -> (w420:string)
          }
          frame False {
            n204 = call <vilib>:"Space Constant.vi"() -> ("String"=w424:string)
            n205 = Concatenate Strings(w426, w425, w424) -> (w423:string)
          }
        }
      }
      n206 = call "FGV FT-IR Diagnosewerte.vi"("Aktionen"=FGV_FT-IR_Diagnose_Aktionen."Lesen") -> ("Temperatur"=w400:dbl)  [unwired: 5 in, 5 out]
      n207 = Number To Fractional String(use system decimal point (T)=FALSE ("Systemdezimalzeichen verwenden (T)"), number=w400, precision (6)=i16 1 ("Genauigkeit (6)")) -> (F-format string=w403:string)  [unwired: 1 in]
      n208 = call <vilib>:"Space Constant.vi"() -> ("String"=w399:string)
      n209 = Concatenate Strings(w406, w399, w403, w394) -> (w409:string)
    }
    frame "AVER" {
      # "OK"
      n210 = call "FGV System Konstanten.vi"("Aktionen"=Aktioen_FGV_System_Konstanten."lesen") -> ("Cluster out"=w428:T28)  [unwired: 6 in, 4 out]
      n211 = Unbundle By Name(w428) -> ("Software Version"=w427:string)
      n212 = call "Zustandsfehlerinformation.vi"("Aktionen"=Aktionen_Zustandsfehlerinformation."OK", "String"=w432) -> ("String"=w431:string)  [unwired: 9 in]
      n213 = call <vilib>:"Space Constant.vi"() -> ("String"=w430:string)
      n214 = Concatenate Strings(w431, w430, w427) -> (w434:string)
    }
    frame "EFDA" {
      # "OK"
      n215 = disable-structure shown="Aktiviert" {
        disable-tunnel: w437 -> [w444 w469]
        disable-tunnel: [w443 w468] -> w436
        disable-tunnel: w435 -> [w442 _]
        frame Disabled {
          n216 = Index Array(array=w442, index #1=2 ("Index"), index #2=3 ("Index")) -> (element #1=w439:string, element #2=w438:string)
          n217 = case shown="\"SEGA\"" w439 {
            tunnel: w444 -> [w446 w457 w467]
            tunnel: [w445 w456 w466] -> w443
            tunnel: w438 -> [_ w449 w459]
            frame " ", Default {
              n218 = call "Zustandsfehlerinformation.vi"("Aktionen"=Aktionen_Zustandsfehlerinformation."Datenfehler", "String"=w446) -> ("String"=w445:string)  [unwired: 9 in]
            }
            frame "SNGA" {
              n219 = Decimal String To Number(string=w449, default (0L)=sgl 0.0) -> (number=w448:sgl)  [unwired: 1 in, 1 out]
              n220 = call "Zustandsfehlerinformation.vi"("Aktionen"=Aktionen_Zustandsfehlerinformation."OK", "String"=w457) -> ("String"=w456:string)  [unwired: 9 in]
              n221 = call "Gespeicherte Werte.vi"("Aktionen"=Aktionen_Gespeicherte_Werte."lesen") -> ("Diverse Werte"=w452:T21)  [unwired: 6 in, 4 out]
              n222 = Bundle By Name(cluster=w452, "Zeit 0-Gas"=w448) -> (w451:T21)
              n223 = call "Gespeicherte Werte.vi"("Aktionen"=Aktionen_Gespeicherte_Werte."Diverse", "Diverse Werte"=w451) -> ()  [unwired: 5 in, 5 out]
            }
            frame "SEGA" {
              n224 = Decimal String To Number(string=w459, default (0L)=sgl 0.0) -> (number=w458:sgl)  [unwired: 1 in, 1 out]
              n225 = call "Zustandsfehlerinformation.vi"("Aktionen"=Aktionen_Zustandsfehlerinformation."OK", "String"=w467) -> ("String"=w466:string)  [unwired: 9 in]
              n226 = call "Gespeicherte Werte.vi"("Aktionen"=Aktionen_Gespeicherte_Werte."lesen") -> ("Diverse Werte"=w462:T21)  [unwired: 6 in, 4 out]
              n227 = Bundle By Name(cluster=w462, "Zeit CalGas"=w458) -> (w461:T21)
              n228 = call "Gespeicherte Werte.vi"("Aktionen"=Aktionen_Gespeicherte_Werte."Diverse", "Diverse Werte"=w461) -> ()  [unwired: 5 in, 5 out]
            }
          }
        }
        frame Enabled {
          n229 = call "Zustandsfehlerinformation.vi"("Aktionen"=Aktionen_Zustandsfehlerinformation."Syntax Error", "String"=w469) -> ("String"=w468:string)  [unwired: 9 in]
        }
      }
    }
    frame "EKFG" {
      # "OK"
      n230 = Index Array(array=w476, index=1 ("Index")) -> (element=w471:string)
      n231 = case shown="\"KV\"" w471 {
        tunnel: w476 -> [_ w481 w495]
        tunnel: [Aktionen_Zustandsfehlerinformation."Syntax Error" ("Aktionen") w478 w492] -> w472
        frame " ", Default {
          # "Befehlskomando NICHT KORREKT!"
        }
        frame "K1" {
          n232 = Delete From Array(array=w481, length=2 ("Länge"), index=0 ("Index")) -> (array with subset deleted=w480:string[])  [unwired: 1 out]
          n233 = Empty Array?(array=w480) -> (empty?=w479:bool)
          n234 = case shown="False" w479 {
            tunnel: w480 -> [w484 _]
            tunnel: [Aktionen_Zustandsfehlerinformation."OK" ("Aktionen") Aktionen_Zustandsfehlerinformation."Datenfehler" ("Aktionen")] -> w478
            frame False {
              n235 = call "AK Namen.vi"("Aktionen"=AK_Namen_Aktionen."EKFG schreiben", "EKFG Liste"=w484) -> ("AK Namen"=w487:string[])  [unwired: 6 in, 3 out]
              n236 = call "AK Namen.vi"("Aktionen"=AK_Namen_Aktionen."EKFG erstellen", "AK Namen"=w487) -> ("AK Namen"=w489:string[])  [unwired: 6 in, 3 out]
              n237 = call "AK Namen.vi"("Aktionen"=AK_Namen_Aktionen."speichern EKFG", "AK Namen"=w489) -> ()  [unwired: 6 in, 4 out]
            }
            frame True {
              # "Fehler mit den Einstell Kommandos"
            }
          }
        }
        frame "KV" {
          n238 = Delete From Array(array=w495, length=3 ("Länge"), index=0 ("Index")) -> (array with subset deleted=w494:string[])  [unwired: 1 out]
          n239 = Empty Array?(array=w494) -> (empty?=w493:bool)
          n240 = case shown="False" w493 {
            tunnel: w494 -> [w500 _]
            tunnel: [Aktionen_Zustandsfehlerinformation."OK" ("Aktionen") Aktionen_Zustandsfehlerinformation."Datenfehler" ("Aktionen")] -> w492
            frame False {
              n241 = call "AK Namen.vi"("Aktionen"=AK_Namen_Aktionen."EKFG schreiben", "EKFG Liste"=w500) -> ("AK Namen"=w503:string[])  [unwired: 6 in, 3 out]
              n242 = call "AK Namen.vi"("Aktionen"=AK_Namen_Aktionen."EKFG erstellen", "KV?"=TRUE, "AK Namen"=w503) -> ()  [unwired: 5 in, 4 out]
            }
            frame True {
              # "Fehler mit den Einstell Kommandos"
            }
          }
        }
      }
      n243 = call "Zustandsfehlerinformation.vi"("Aktionen"=w472, "String"=w475) -> ("String"=w474:string)  [unwired: 9 in]
    }
    frame "EMET" {
      # "OK"
      n244 = Index Array(array=w507, index=1 ("Index")) -> (element=w511:string)
      n245 = Equal?(x=w511, y="K0") -> (x = y?=w509:bool)
      n246 = case shown="True" w509 {
        tunnel: w507 -> [_ w517]
        tunnel: [Aktionen_Zustandsfehlerinformation."Syntax Error" ("Aktionen") w514] -> w508
        frame False {
          # "Befehlskomando NICHT KORREKT!"
        }
        frame True {
          n247 = Delete From Array(array=w517, length=2 ("Länge"), index=0 ("Index")) -> (array with subset deleted=w516:string[])  [unwired: 1 out]
          n248 = Empty Array?(array=w516) -> (empty?=w515:bool)
          n249 = case shown="False" w515 {
            tunnel: w516 -> [w521 _]
            tunnel: [w522 Aktionen_Zustandsfehlerinformation."Datenfehler" ("Aktionen")] -> w514
            frame False {
              n250 = Index Array(array=w521) -> (element=w520:string)  [unwired: 1 in]
              n251 = case shown="\"CNG\"" w520 {
                tunnel: [Aktionen_Zustandsfehlerinformation."OK" ("Aktionen") Aktionen_Zustandsfehlerinformation."Syntax Error" ("Aktionen") Aktionen_Zustandsfehlerinformation."OK" ("Aktionen") Aktionen_Zustandsfehlerinformation."OK" ("Aktionen")] -> w522
                frame "CNG" {
                  n252 = call "FGV Rezepte wechseln.vi"("AK/man"=AK-manuell."CNG", "Aktion"=Aktion_FGV_Rezepte_wechseln."AK/Man") -> ("error out"=w525:errorcluster)  [unwired: 7 in, 6 out]
                  n253 = flat-sequence {
                    tunnel: w525 -> [_]
                    frame #0 {
                      n254 = vi-ref "FT-IR.lvlib:TOOLweb Interface.lvlib:TOOLweb Rezept wechseln.vi"() -> (w527:refnum<vi>)
                      n255 = call "VI Pop Up.vi"("VI Referenz"=w527) -> ()  [unwired: 10 in, 1 out]
                    }
                  }
                }
                frame "0", Default {
                }
                frame "DIESEL" {
                  n256 = call "FGV Rezepte wechseln.vi"("AK/man"=AK-manuell."Diesel", "Aktion"=Aktion_FGV_Rezepte_wechseln."AK/Man") -> ("error out"=w531:errorcluster)  [unwired: 7 in, 6 out]
                  n257 = flat-sequence {
                    tunnel: w531 -> [_]
                    frame #0 {
                      n258 = vi-ref "FT-IR.lvlib:TOOLweb Interface.lvlib:TOOLweb Rezept wechseln.vi"() -> (w533:refnum<vi>)
                      n259 = call "VI Pop Up.vi"("VI Referenz"=w533) -> ()  [unwired: 10 in, 1 out]
                    }
                  }
                }
                frame "GASOLINE" {
                  n260 = call "FGV Rezepte wechseln.vi"("AK/man"=AK-manuell."Gasoline", "Aktion"=Aktion_FGV_Rezepte_wechseln."AK/Man") -> ("error out"=w536:errorcluster)  [unwired: 7 in, 6 out]
                  n261 = flat-sequence {
                    tunnel: w536 -> [_]
                    frame #0 {
                      n262 = vi-ref "FT-IR.lvlib:TOOLweb Interface.lvlib:TOOLweb Rezept wechseln.vi"() -> (w538:refnum<vi>)
                      n263 = call "VI Pop Up.vi"("VI Referenz"=w538) -> ()  [unwired: 10 in, 1 out]
                    }
                  }
                }
              }
            }
            frame True {
              # "Fehler mit den Einstell Kommandos"
            }
          }
        }
      }
      n264 = call "Zustandsfehlerinformation.vi"("Aktionen"=w508, "String"=w506) -> ("String"=w505:string)  [unwired: 9 in]
    }
    frame "SARA" {
      n265 = call "Zustandsfehlerinformation.vi"("Aktionen"=Aktionen_Zustandsfehlerinformation."OK", "String"=w541) -> ("String"=w540:string)  [unwired: 9 in]
    }
    frame "SARE" {
      n266 = call "Zustandsfehlerinformation.vi"("Aktionen"=Aktionen_Zustandsfehlerinformation."OK", "String"=w544) -> ("String"=w543:string)  [unwired: 9 in]
    }
    frame "SATK" {
      n267 = call "Setze Zustand.vi"("AK Befehl"=w547, "Zustand"=Zustaende."Kalibrieren") -> ("Antwort String"=w546:string)  [unwired: 8 in, 1 out]
    }
    frame "SECO" {
      # "OK"
      n268 = call "Setze Zustand.vi"("AK Befehl"=w551, "Zustand"=Zustaende."Eco") -> ("Antwort String"=w550:string)  [unwired: 8 in, 1 out]
    }
    frame "SEGA" {
      n269 = call "FGV-Funktionstasten.vi"("Aktion"=Funktionstasten-Aktion."Lesen") -> ("Betriebsart"=w556:T17)  [unwired: 7 in, 7 out]
      n270 = Equal?(x=w556, y=Betriebsart."Remote" ("Betriebsart")) -> (x = y?=w557:bool)
      n271 = case shown="True" w557 {
        tunnel: w553 -> [w559 w562]
        tunnel: [w558 w561] -> w552
        frame False {
          n272 = call "Zustandsfehlerinformation.vi"("Aktionen"=Aktionen_Zustandsfehlerinformation."Offline", "String"=w559) -> ("String"=w558:string)  [unwired: 9 in]
        }
        frame True {
          n273 = disable-structure shown="Deaktiviert" {
            frame Disabled {
              n274 = call "Gespeicherte Werte.vi"("Aktionen"=Aktionen_Gespeicherte_Werte."lesen") -> ("Diverse Werte"=w564:T21)  [unwired: 6 in, 4 out]
              n275 = Unbundle By Name(w564) -> ()  [unwired: 1 out]
            }
            frame Enabled {
            }
          }
          n276 = call "Setze Zustand.vi"("AK Befehl"=w562, "Zustand"=Zustaende."Cal-Gas") -> ("Antwort String"=w561:string)  [unwired: 8 in, 1 out]
        }
      }
    }
    frame "SEKA" {
      n277 = call "Zustandsfehlerinformation.vi"("Aktionen"=Aktionen_Zustandsfehlerinformation."OK", "String"=w567) -> ("String"=w566:string)  [unwired: 9 in]
    }
    frame "SEMB" {
      # "OK"
      n278 = call "FGV-Funktionstasten.vi"("Aktion"=Funktionstasten-Aktion."Lesen") -> ("Betriebsart"=w574:T17)  [unwired: 7 in, 7 out]
      n279 = Equal?(x=w574, y=Betriebsart."Remote" ("Betriebsart")) -> (x = y?=w575:bool)
      n280 = case shown="True" w575 {
        tunnel: w571 -> [w577 w589]
        tunnel: [w576 w588] -> w570
        tunnel: w569 -> [_ w587]
        frame False {
          n281 = call "Zustandsfehlerinformation.vi"("Aktionen"=Aktionen_Zustandsfehlerinformation."Offline", "String"=w577) -> ("String"=w576:string)  [unwired: 9 in]
        }
        frame True {
          n282 = Index Array(array=w587, index=2 ("Index")) -> (element=w580:string)
          n283 = call "Zustandsfehlerinformation.vi"("Aktionen"=Aktionen_Zustandsfehlerinformation."OK", "String"=w589) -> ("String"=w588:string)  [unwired: 9 in]
          n284 = Decimal String To Number(string=w580, offset=1 ("Offset (0)")) -> (number=w579:i32)  [unwired: 1 in, 1 out]
          n285 = call "Gespeicherte Werte.vi"("Aktionen"=Aktionen_Gespeicherte_Werte."lesen") -> ("Diverse Werte"=w582:T21)  [unwired: 6 in, 4 out]
          n286 = Bundle By Name(cluster=w582, "Kalibriergaseingang"=w579) -> (w581:T21)
          n287 = call "Gespeicherte Werte.vi"("Aktionen"=Aktionen_Gespeicherte_Werte."Diverse", "Diverse Werte"=w581) -> ()  [unwired: 5 in, 5 out]
        }
      }
    }
    frame "SENT" {
      n288 = call "FGV-Funktionstasten.vi"("Aktion"=Funktionstasten-Aktion."Lesen") -> ("Betriebsart"=w596:T17)  [unwired: 7 in, 7 out]
      n289 = Equal?(x=w596, y=Betriebsart."Remote" ("Betriebsart")) -> (x = y?=w597:bool)
      n290 = case shown="True" w597 {
        tunnel: w593 -> [w599 w616]
        tunnel: [w598 w615] -> w592
        tunnel: w591 -> [_ w601]
        frame False {
          n291 = call "Zustandsfehlerinformation.vi"("Aktionen"=Aktionen_Zustandsfehlerinformation."Offline", "String"=w599) -> ("String"=w598:string)  [unwired: 9 in]
        }
        frame True {
          n292 = Array Size(array=w601) -> (size(s)=w603:i32)
          n293 = Greater?(x=w603, y=3) -> (0:w605:bool)
          n294 = Select(t=3, s=w605, f=2 ("Index")) -> (s? t:f=w608:i32)
          n295 = Index Array(array=w601, index=w608) -> (element=w602:string)
          n296 = call "Zustandsfehlerinformation.vi"("Aktionen"=Aktionen_Zustandsfehlerinformation."OK", "String"=w616) -> ("String"=w615:string)  [unwired: 9 in]
          n297 = Decimal String To Number(string=w602) -> (number=w609:i32)  [unwired: 2 in, 1 out]
          n298 = call "FGV-Funktionstasten.vi"("Samplepoint"=w609, "Aktion"=Funktionstasten-Aktion."Samplepoint") -> ()  [unwired: 6 in, 8 out]
          n299 = call "Gespeicherte Werte.vi"("Aktionen"=Aktionen_Gespeicherte_Werte."lesen") -> ("Diverse Werte"=w612:T21)  [unwired: 6 in, 4 out]
          n300 = Bundle By Name(cluster=w612, "SamplePoint"=w609) -> (w611:T21)
          n301 = call "Gespeicherte Werte.vi"("Aktionen"=Aktionen_Gespeicherte_Werte."Diverse", "Diverse Werte"=w611) -> ()  [unwired: 5 in, 5 out]
        }
      }
    }
    frame "SINT" {
      n302 = call "Setze Zustand.vi"("AK Befehl"=w620, "Zustand"=Zustaende."Messen") -> ("Antwort String"=w619:string)  [unwired: 8 in, 1 out]
    }
    frame "SLCR" {
      # "OK"
      n303 = Index Array(array=w630, index=1 ("Index")) -> (element=w628:string)
      n304 = call "FGV-Funktionstasten.vi"("Aktion"=Funktionstasten-Aktion."Lesen") -> ("Busy"=w621:bool, "Betriebsart"=w627:T17)  [unwired: 7 in, 6 out]
      n305 = Equal?(x=w627, y=Betriebsart."Remote" ("Betriebsart")) -> (x = y?=w624:bool)
      n306 = case shown="False" w624 {
        tunnel: w628 -> [_ w637]
        tunnel: w623 -> [w632 w636]
        tunnel: [w631 w635] -> w622
        tunnel: w621 -> [_ w634]
        frame False {
          n307 = call "Zustandsfehlerinformation.vi"("Aktionen"=Aktionen_Zustandsfehlerinformation."Offline", "String"=w632) -> ("String"=w631:string)  [unwired: 9 in]
        }
        frame True {
          n308 = case shown="True" w634 {
            tunnel: w637 -> [w640 _]
            tunnel: w636 -> [w639 w654]
            tunnel: [w638 w653] -> w635
            frame False {
              n309 = case shown="\"K0\"" w640 {
                tunnel: w639 -> [w642 w649]
                tunnel: [w641 w648] -> w638
                frame "Standard", Default {
                  n310 = call "Zustandsfehlerinformation.vi"("Aktionen"=Aktionen_Zustandsfehlerinformation."Syntax Error", "String"=w642) -> ("String"=w641:string)  [unwired: 9 in]
                }
                frame "K0" {
                  n311 = call "FGV Automatic start.vi"("Aktion"=Aktion_FGV_Automatic_start."Seite merken") -> ("error out"=w645:errorcluster)  [unwired: 12 in, 2 out]
                  n312 = flat-sequence {
                    tunnel: w645 -> [w652]
                    tunnel: [w652] -> w644
                    frame #0 {
                      n313 = call "Bildwechsel.vi"("nächstes Bild"=Bild-Auswahl."EPA Dichtheitstest") -> ()  [unwired: 9 in, 2 out]
                    }
                  }
                  n314 = call "Zustandsfehlerinformation.vi"("Aktionen"=Aktionen_Zustandsfehlerinformation."OK", "String"=w649) -> ("String"=w648:string)  [unwired: 9 in]
                  n315 = call "FGV Automatic start.vi"("error in (no error)"=w644, "Aktion"=Aktion_FGV_Automatic_start."Test starten aktiv") -> ()  [unwired: 11 in, 3 out]
                }
              }
            }
            frame True {
              n316 = call "Zustandsfehlerinformation.vi"("Aktionen"=Aktionen_Zustandsfehlerinformation."Busy", "String"=w654) -> ("String"=w653:string)  [unwired: 9 in]
            }
          }
        }
      }
    }
    frame "SLEC" {
      n317 = call "Setze Zustand.vi"("AK Befehl"=w659, "Zustand"=Zustaende."Standby") -> ("Antwort String"=w658:string, "Busy"=w656:bool)  [unwired: 8 in]
      n318 = case shown="False" w656 {
        frame False {
          n319 = vi-ref "Dichtheitstest.vi"() -> (w660:refnum<vi>)
          n320 = call "VI Pop Up.vi"("VI Referenz"=w660) -> ()  [unwired: 10 in, 1 out]
        }
        frame True {
          # "Busy"
        }
      }
    }
    frame "SMAN" {
      n321 = call "FGV-Funktionstasten.vi"("Aktion"=Funktionstasten-Aktion."Lesen") -> ("Betriebsart"=w666:T17)  [unwired: 7 in, 7 out]
      n322 = Equal?(x=w666, y=Betriebsart."Remote" ("Betriebsart")) -> (x = y?=w663:bool)
      n323 = case shown="True" w663 {
        tunnel: w662 -> [w669 w672]
        tunnel: [w667 w671] -> w661
        frame False {
          n324 = call "Zustandsfehlerinformation.vi"("Aktionen"=Aktionen_Zustandsfehlerinformation."Offline", "String"=w669) -> ("String"=w667:string)  [unwired: 9 in]
        }
        frame True {
          n325 = call "Zustandsfehlerinformation.vi"("Aktionen"=Aktionen_Zustandsfehlerinformation."OK", "String"=w672) -> ("String"=w671:string)  [unwired: 9 in]
          n326 = call "FGV-Funktionstasten.vi"("Aktion"=Funktionstasten-Aktion."Manuell") -> ()  [unwired: 7 in, 8 out]
        }
      }
    }
    frame "SMGA" {
      n327 = call "Setze Zustand.vi"("AK Befehl"=w676, "Zustand"=Zustaende."Messen") -> ("Antwort String"=w675:string)  [unwired: 8 in, 1 out]
    }
    frame "SNGA" {
      n328 = call "Setze Zustand.vi"("AK Befehl"=w679, "Zustand"=Zustaende."0-Gas") -> ("Antwort String"=w678:string)  [unwired: 8 in, 1 out]
    }
    frame "SNGF" {
      # "OK"
      n329 = call "Setze Zustand.vi"("Befehl nicht vorhanden!"=TRUE, "AK Befehl"=w683, "Zustand"=Zustaende."Standby") -> ("Antwort String"=w682:string)  [unwired: 7 in, 1 out]
    }
    frame "SNKA" {
      n330 = call "Zustandsfehlerinformation.vi"("Aktionen"=Aktionen_Zustandsfehlerinformation."OK", "String"=w685) -> ("String"=w684:string)  [unwired: 9 in]
    }
    frame "SPAU" {
      # "OK"
      n331 = call "Setze Zustand.vi"("AK Befehl"=w689, "Zustand"=Zustaende."Pause") -> ("Antwort String"=w688:string)  [unwired: 8 in, 1 out]
    }
    frame "SREM" {
      # "OK"
      n332 = call "Zustandsfehlerinformation.vi"("Aktionen"=Aktionen_Zustandsfehlerinformation."OK", "String"=w691) -> ("String"=w690:string)  [unwired: 9 in]
      n333 = call "FGV-Funktionstasten.vi"("Aktion"=Funktionstasten-Aktion."Remote") -> ()  [unwired: 7 in, 8 out]
    }
    frame "SRES" {
      n334 = call "Zustandsfehlerinformation.vi"("Aktionen"=Aktionen_Zustandsfehlerinformation."OK", "String"=w695) -> ("String"=w694:string)  [unwired: 9 in]
    }
    frame "SRUC" {
      # "OK"
      n335 = Index Array(array=w698, index=2 ("Index")) -> (element=w700:string)
      n336 = Decimal String To Number(string=w700) -> (number=w701:i32)  [unwired: 2 in, 1 out]
      n337 = Divide(x=w701, y=10) -> (x/y=w703:dbl)
      n338 = To Single Precision Float(number=w703) -> (single precision float=w697:sgl)
      n339 = call "Setze Zustand.vi"("Zeit"=w697, "AK Befehl"=w706, "Zustand"=Zustaende."Spülen Filter") -> ("Antwort String"=w705:string)  [unwired: 7 in, 1 out]
    }
    frame "SRUK" {
      # "OK"
      n340 = Index Array(array=w707, index=2 ("Index")) -> (element=w710:string)
      n341 = Decimal String To Number(string=w710) -> (number=w711:i32)  [unwired: 2 in, 1 out]
      n342 = Divide(x=w711, y=10) -> (x/y=w713:dbl)
      n343 = To Single Precision Float(number=w713) -> (single precision float=w708:sgl)
      n344 = call "Setze Zustand.vi"("Zeit"=w708, "AK Befehl"=w716, "Zustand"=Zustaende."Spülen Filter") -> ("Antwort String"=w715:string)  [unwired: 7 in, 1 out]
    }
    frame "SSPL" {
      # "OK"
      n345 = Index Array(array=w718, index=2 ("Index")) -> (element=w720:string)
      n346 = Decimal String To Number(string=w720) -> (number=w721:i32)  [unwired: 2 in, 1 out]
      n347 = Divide(x=w721, y=10) -> (x/y=w723:dbl)
      n348 = To Single Precision Float(number=w723) -> (single precision float=w717:sgl)
      n349 = call "Setze Zustand.vi"("Zeit"=w717, "AK Befehl"=w726, "Zustand"=Zustaende."Spülen Leitung") -> ("Antwort String"=w725:string)  [unwired: 7 in, 1 out]
    }
    frame "SSPR" {
      # "OK"
      n350 = call "Setze Zustand.vi"("Befehl nicht vorhanden!"=TRUE, "AK Befehl"=w730, "Zustand"=Zustaende."Standby") -> ("Antwort String"=w729:string)  [unwired: 7 in, 1 out]
    }
    frame "STBY" {
      # "OK"
      n351 = call "Setze Zustand.vi"("AK Befehl"=w733, "Zustand"=Zustaende."Standby") -> ("Antwort String"=w732:string)  [unwired: 8 in, 1 out]
    }
    frame "STRG" {
      n352 = call "FGV-Funktionstasten.vi"("Aktion"=Funktionstasten-Aktion."Lesen") -> ("Betriebsart"=w739:T17)  [unwired: 7 in, 7 out]
      n353 = Equal?(x=w739, y=Betriebsart."Remote" ("Betriebsart")) -> (x = y?=w740:bool)
      n354 = case shown="True" w740 {
        tunnel: w736 -> [w742 w749]
        tunnel: [w741 w748] -> w735
        tunnel: w734 -> [_ w747]
        frame False {
          n355 = call "Zustandsfehlerinformation.vi"("Aktionen"=Aktionen_Zustandsfehlerinformation."Offline", "String"=w742) -> ("String"=w741:string)  [unwired: 9 in]
        }
        frame True {
          n356 = Index Array(array=w747, index=2 ("Index")) -> (element=w745:string)
          n357 = call "Zustandsfehlerinformation.vi"("Aktionen"=Aktionen_Zustandsfehlerinformation."OK", "String"=w749) -> ("String"=w748:string)  [unwired: 9 in]
          n358 = Empty String/Path?(string/path=w745) -> (empty?=w744:bool)
          n359 = case shown="False" w744 {
            tunnel: w745 -> [w756 _]
            frame False {
              n360 = Decimal String To Number(string=w756) -> (number=w753:i32)  [unwired: 2 in, 1 out]
              n361 = call "FGV Trigger.vi"("Aktion"=Aktionen_Trigger."lesen") -> ("Triggerereignis neu"=w752:T29)  [unwired: 7 in, 3 out]
              n362 = Bundle By Name(cluster=w752, "Trigger verwenden"=w753) -> (w751:T29)
              n363 = call "FGV Trigger.vi"("Aktion"=Aktionen_Trigger."ALLE schreiben", "Triggerereignis"=w751) -> ()  [unwired: 6 in, 4 out]
            }
            frame True {
            }
          }
        }
      }
    }
    frame "SUGR" {
      n364 = call "Setze Zustand.vi"("AK Befehl"=w758, "Zustand"=Zustaende."Kalibrieren") -> ("Antwort String"=w757:string)  [unwired: 8 in, 1 out]
    }
  }
  "String für schreiben" <- w5
